vi "GetPirticleResultNames.vi"(7 "ProjectName":string="Prj", 9 "Selected Particle Report":T1(array[cluster])=[{"Area"=25.0, "Number of Holes"=0.0, "Bounding Rect"={"Left"=86.0, "Top"=0.0, "Right"=95.0, "Bottom"=7.0}, "Center of Mass"={"X"=89.88, "Y"=2.56}, "Orientation"=35.64802944169076, "Dimensions"={"Width"=9.0, "Height"=7.0}}, {"Area"=86262.0, "Number of Holes"=23.0, "Bounding Rect"={"Left"=0.0, "Top"=0.0, "Right"=463.0, "Bottom"=400.0}, "Center of Mass"={"X"=231.6348565996615, "Y"=215.4975423709165}, "Orientation"=163.33264135410136, "Dimensions"={"Width"=463.0, "Height"=400.0}}, {"Area"=1.0, "Number of Holes"=0.0, "Bounding Rect"={"Left"=412.0, "Top"=1.0, "Right"=413.0, "Bottom"=2.0}, "Center of Mass"={"X"=412.0, "Y"=1.0}, "Orientation"=-0.0, "Dimensions"={"Width"=1.0, "Height"=1.0}}, {"Area"=764.0, "Number of Holes"=1.0, "Bounding Rect"={"Left"=400.0, "Top"=1.0, "Right"=429.0, "Bottom"=38.0}, "Center of Mass"={"X"=414.1609947643979, "Y"=19.994764397905758}, "Orientation"=91.15464026101695, "Dimensions"={"Width"=29.0, "Height"=37.0}}, {"Area"=59.0, "Number of Holes"=0.0, "Bounding Rect"={"Left"=310.0, "Top"=6.0, "Right"=340.0, "Bottom"=29.0}, "Center of Mass"={"X"=326.50847457627117, "Y"=15.610169491525424}, "Orientation"=141.9692279302436, "Dimensions"={"Width"=30.0, "Height"=23.0}}, {"Area"=11.0, "Number of Holes"=0.0, "Bounding Rect"={"Left"=0.0, "Top"=7.0, "Right"=8.0, "Bottom"=12.0}, "Center of Mass"={"X"=3.090909090909091, "Y"=9.0}, "Orientation"=154.0962999034186, "Dimensions"={"Width"=8.0, "Height"=5.0}}, {"Area"=8.0, "Number of Holes"=0.0, "Bounding Rect"={"Left"=10.0, "Top"=12.0, "Right"=18.0, "Bottom"=15.0}, "Center of Mass"={"X"=13.5, "Y"=13.125}, "Orientation"=161.9863133074482, "Dimensions"={"Width"=8.0, "Height"=3.0}}, {"Area"=2191.0, "Number of Holes"=0.0, "Bounding Rect"={"Left"=108.0, "Top"=12.0, "Right"=160.0, "Bottom"=73.0}, "Center of Mass"={"X"=132.4596074851666, "Y"=44.30716567777271}, "Orientation"=94.97370367521454, "Dimensions"={"Width"=52.0, "Height"=61.0}}, {"Area"=18.0, "Number of Holes"=0.0, "Bounding Rect"={"Left"=136.0, "Top"=12.0, "Right"=150.0, "Bottom"=18.0}, "Center of Mass"={"X"=142.94444444444446, "Y"=13.833333333333334}, "Orientation"=159.1562056734768, "Dimensions"={"Width"=14.0, "Height"=6.0}}, {"Area"=4659.0, "Number of Holes"=2.0, "Bounding Rect"={"Left"=266.0, "Top"=12.0, "Right"=345.0, "Bottom"=101.0}, "Center of Mass"={"X"=303.5157759175789, "Y"=58.89869070616012}, "Orientation"=93.68626534635163, "Dimensions"={"Width"=79.0, "Height"=89.0}}, {"Area"=12.0, "Number of Holes"=0.0, "Bounding Rect"={"Left"=19.0, "Top"=14.0, "Right"=29.0, "Bottom"=17.0}, "Center of Mass"={"X"=23.083333333333332, "Y"=15.416666666666666}, "Orientation"=169.41797481154816, "Dimensions"={"Width"=10.0, "Height"=3.0}}, {"Area"=6.0, "Number of Holes"=0.0, "Bounding Rect"={"Left"=32.0, "Top"=17.0, "Right"=38.0, "Bottom"=18.0}, "Center of Mass"={"X"=34.5, "Y"=17.0}, "Orientation"=-0.0, "Dimensions"={"Width"=6.0, "Height"=1.0}}, {"Area"=1.0, "Number of Holes"=0.0, "Bounding Rect"={"Left"=40.0, "Top"=17.0, "Right"=41.0, "Bottom"=18.0}, "Center of Mass"={"X"=40.0, "Y"=17.0}, "Orientation"=-0.0, "Dimensions"={"Width"=1.0, "Height"=1.0}}, {"Area"=1.0, "Number of Holes"=0.0, "Bounding Rect"={"Left"=326.0, "Top"=23.0, "Right"=327.0, "Bottom"=24.0}, "Center of Mass"={"X"=326.0, "Y"=23.0}, "Orientation"=-0.0, "Dimensions"={"Width"=1.0, "Height"=1.0}}, {"Area"=72.0, "Number of Holes"=2.0, "Bounding Rect"={"Left"=388.0, "Top"=35.0, "Right"=410.0, "Bottom"=55.0}, "Center of Mass"={"X"=397.8888888888889, "Y"=46.52777777777778}, "Orientation"=136.8853757704328, "Dimensions"={"Width"=22.0, "Height"=20.0}}, {"Area"=2.0, "Number of Holes"=0.0, "Bounding Rect"={"Left"=342.0, "Top"=36.0, "Right"=343.0, "Bottom"=38.0}, "Center of Mass"={"X"=342.0, "Y"=36.5}, "Orientation"=90.0, "Dimensions"={"Width"=1.0, "Height"=2.0}}, {"Area"=1.0, "Number of Holes"=0.0, "Bounding Rect"={"Left"=396.0, "Top"=49.0, "Right"=397.0, "Bottom"=50.0}, "Center of Mass"={"X"=396.0, "Y"=49.0}, "Orientation"=-0.0, "Dimensions"={"Width"=1.0, "Height"=1.0}}, {"Area"=2.0, "Number of Holes"=0.0, "Bounding Rect"={"Left"=411.0, "Top"=54.0, "Right"=413.0, "Bottom"=55.0}, "Center of Mass"={"X"=411.5, "Y"=54.0}, "Orientation"=-0.0, "Dimensions"={"Width"=2.0, "Height"=1.0}}, {"Area"=86.0, "Number of Holes"=0.0, "Bounding Rect"={"Left"=457.0, "Top"=74.0, "Right"=463.0, "Bottom"=96.0}, "Center of Mass"={"X"=460.2674418604651, "Y"=84.55813953488372}, "Orientation"=89.65892383367937, "Dimensions"={"Width"=6.0, "Height"=22.0}}, {"Area"=1300.0, "Number of Holes"=0.0, "Bounding Rect"={"Left"=30.0, "Top"=82.0, "Right"=67.0, "Bottom"=127.0}, "Center of Mass"={"X"=48.050769230769234, "Y"=104.12153846153846}, "Orientation"=84.17144755534598, "Dimensions"={"Width"=37.0, "Height"=45.0}}, {"Area"=1.0, "Number of Holes"=0.0, "Bounding Rect"={"Left"=450.0, "Top"=105.0, "Right"=451.0, "Bottom"=106.0}, "Center of Mass"={"X"=450.0, "Y"=105.0}, "Orientation"=-0.0, "Dimensions"={"Width"=1.0, "Height"=1.0}}, {"Area"=3.0, "Number of Holes"=0.0, "Bounding Rect"={"Left"=243.0, "Top"=124.0, "Right"=245.0, "Bottom"=126.0}, "Center of Mass"={"X"=243.66666666666666, "Y"=124.33333333333333}, "Orientation"=135.00000000000014, "Dimensions"={"Width"=2.0, "Height"=2.0}}, {"Area"=28.0, "Number of Holes"=0.0, "Bounding Rect"={"Left"=271.0, "Top"=127.0, "Right"=293.0, "Bottom"=136.0}, "Center of Mass"={"X"=281.39285714285717, "Y"=131.39285714285714}, "Orientation"=158.88118737593115, "Dimensions"={"Width"=22.0, "Height"=9.0}}, {"Area"=4.0, "Number of Holes"=0.0, "Bounding Rect"={"Left"=250.0, "Top"=128.0, "Right"=253.0, "Bottom"=130.0}, "Center of Mass"={"X"=251.0, "Y"=128.5}, "Orientation"=148.282525588539, "Dimensions"={"Width"=3.0, "Height"=2.0}}, {"Area"=4.0, "Number of Holes"=0.0, "Bounding Rect"={"Left"=255.0, "Top"=132.0, "Right"=258.0, "Bottom"=134.0}, "Center of Mass"={"X"=256.0, "Y"=132.5}, "Orientation"=148.282525588539, "Dimensions"={"Width"=3.0, "Height"=2.0}}, {"Area"=2.0, "Number of Holes"=0.0, "Bounding Rect"={"Left"=260.0, "Top"=136.0, "Right"=262.0, "Bottom"=138.0}, "Center of Mass"={"X"=260.5, "Y"=136.5}, "Orientation"=135.0, "Dimensions"={"Width"=2.0, "Height"=2.0}}, {"Area"=1.0, "Number of Holes"=0.0, "Bounding Rect"={"Left"=300.0, "Top"=136.0, "Right"=301.0, "Bottom"=137.0}, "Center of Mass"={"X"=300.0, "Y"=136.0}, "Orientation"=-0.0, "Dimensions"={"Width"=1.0, "Height"=1.0}}, {"Area"=6.0, "Number of Holes"=0.0, "Bounding Rect"={"Left"=263.0, "Top"=139.0, "Right"=269.0, "Bottom"=145.0}, "Center of Mass"={"X"=265.5, "Y"=141.5}, "Orientation"=135.0, "Dimensions"={"Width"=6.0, "Height"=6.0}}, {"Area"=4.0, "Number of Holes"=0.0, "Bounding Rect"={"Left"=296.0, "Top"=139.0, "Right"=299.0, "Bottom"=141.0}, "Center of Mass"={"X"=297.25, "Y"=139.25}, "Orientation"=161.56505117707798, "Dimensions"={"Width"=3.0, "Height"=2.0}}, {"Area"=1.0, "Number of Holes"=0.0, "Bounding Rect"={"Left"=269.0, "Top"=146.0, "Right"=270.0, "Bottom"=147.0}, "Center of Mass"={"X"=269.0, "Y"=146.0}, "Orientation"=-0.0, "Dimensions"={"Width"=1.0, "Height"=1.0}}, {"Area"=3.0, "Number of Holes"=0.0, "Bounding Rect"={"Left"=271.0, "Top"=148.0, "Right"=273.0, "Bottom"=151.0}, "Center of Mass"={"X"=271.3333333333333, "Y"=149.0}, "Orientation"=118.15496623701016, "Dimensions"={"Width"=2.0, "Height"=3.0}}, {"Area"=2795.0, "Number of Holes"=2.0, "Bounding Rect"={"Left"=375.0, "Top"=149.0, "Right"=427.0, "Bottom"=220.0}, "Center of Mass"={"X"=400.8608228980322, "Y"=184.37352415026834}, "Orientation"=84.46336335814708, "Dimensions"={"Width"=52.0, "Height"=71.0}}, {"Area"=6024.0, "Number of Holes"=9.0, "Bounding Rect"={"Left"=176.0, "Top"=152.0, "Right"=254.0, "Bottom"=252.0}, "Center of Mass"={"X"=211.63097609561754, "Y"=201.42861885790174}, "Orientation"=84.84991716022375, "Dimensions"={"Width"=78.0, "Height"=100.0}}, {"Area"=1.0, "Number of Holes"=0.0, "Bounding Rect"={"Left"=275.0, "Top"=154.0, "Right"=276.0, "Bottom"=155.0}, "Center of Mass"={"X"=275.0, "Y"=154.0}, "Orientation"=-0.0, "Dimensions"={"Width"=1.0, "Height"=1.0}}, {"Area"=2.0, "Number of Holes"=0.0, "Bounding Rect"={"Left"=462.0, "Top"=209.0, "Right"=463.0, "Bottom"=211.0}, "Center of Mass"={"X"=462.0, "Y"=209.5}, "Orientation"=90.0, "Dimensions"={"Width"=1.0, "Height"=2.0}}, {"Area"=1.0, "Number of Holes"=0.0, "Bounding Rect"={"Left"=460.0, "Top"=214.0, "Right"=461.0, "Bottom"=215.0}, "Center of Mass"={"X"=460.0, "Y"=214.0}, "Orientation"=-0.0, "Dimensions"={"Width"=1.0, "Height"=1.0}}, {"Area"=2.0, "Number of Holes"=0.0, "Bounding Rect"={"Left"=459.0, "Top"=216.0, "Right"=460.0, "Bottom"=218.0}, "Center of Mass"={"X"=459.0, "Y"=216.5}, "Orientation"=90.0, "Dimensions"={"Width"=1.0, "Height"=2.0}}, {"Area"=3.0, "Number of Holes"=0.0, "Bounding Rect"={"Left"=249.0, "Top"=220.0, "Right"=251.0, "Bottom"=223.0}, "Center of Mass"={"X"=249.66666666666666, "Y"=221.0}, "Orientation"=61.84503376298985, "Dimensions"={"Width"=2.0, "Height"=3.0}}, {"Area"=1243.0, "Number of Holes"=2.0, "Bounding Rect"={"Left"=26.0, "Top"=222.0, "Right"=62.0, "Bottom"=266.0}, "Center of Mass"={"X"=43.17940466613033, "Y"=243.51729686242962}, "Orientation"=85.94368880614128, "Dimensions"={"Width"=36.0, "Height"=44.0}}, {"Area"=3.0, "Number of Holes"=0.0, "Bounding Rect"={"Left"=248.0, "Top"=224.0, "Right"=250.0, "Bottom"=227.0}, "Center of Mass"={"X"=248.33333333333334, "Y"=225.0}, "Orientation"=61.84503376298985, "Dimensions"={"Width"=2.0, "Height"=3.0}}, {"Area"=1.0, "Number of Holes"=0.0, "Bounding Rect"={"Left"=62.0, "Top"=237.0, "Right"=63.0, "Bottom"=238.0}, "Center of Mass"={"X"=62.0, "Y"=237.0}, "Orientation"=-0.0, "Dimensions"={"Width"=1.0, "Height"=1.0}}, {"Area"=1.0, "Number of Holes"=0.0, "Bounding Rect"={"Left"=63.0, "Top"=241.0, "Right"=64.0, "Bottom"=242.0}, "Center of Mass"={"X"=63.0, "Y"=241.0}, "Orientation"=-0.0, "Dimensions"={"Width"=1.0, "Height"=1.0}}, {"Area"=25.0, "Number of Holes"=0.0, "Bounding Rect"={"Left"=60.0, "Top"=277.0, "Right"=78.0, "Bottom"=285.0}, "Center of Mass"={"X"=68.52, "Y"=279.96}, "Orientation"=21.66201240397291, "Dimensions"={"Width"=18.0, "Height"=8.0}}, {"Area"=2.0, "Number of Holes"=0.0, "Bounding Rect"={"Left"=57.0, "Top"=285.0, "Right"=59.0, "Bottom"=287.0}, "Center of Mass"={"X"=57.5, "Y"=285.5}, "Orientation"=45.0, "Dimensions"={"Width"=2.0, "Height"=2.0}}, {"Area"=1575.0, "Number of Holes"=0.0, "Bounding Rect"={"Left"=302.0, "Top"=285.0, "Right"=345.0, "Bottom"=337.0}, "Center of Mass"={"X"=321.4095238095238, "Y"=308.74603174603175}, "Orientation"=73.7943685874199, "Dimensions"={"Width"=43.0, "Height"=52.0}}, {"Area"=4853.0, "Number of Holes"=6.0, "Bounding Rect"={"Left"=54.0, "Top"=304.0, "Right"=130.0, "Bottom"=388.0}, "Center of Mass"={"X"=91.93962497424273, "Y"=344.35854110859265}, "Orientation"=86.14198788768665, "Dimensions"={"Width"=76.0, "Height"=84.0}}, {"Area"=28.0, "Number of Holes"=0.0, "Bounding Rect"={"Left"=323.0, "Top"=332.0, "Right"=338.0, "Bottom"=341.0}, "Center of Mass"={"X"=330.57142857142856, "Y"=336.64285714285717}, "Orientation"=29.47782205630064, "Dimensions"={"Width"=15.0, "Height"=9.0}}, {"Area"=3.0, "Number of Holes"=0.0, "Bounding Rect"={"Left"=312.0, "Top"=366.0, "Right"=315.0, "Bottom"=367.0}, "Center of Mass"={"X"=313.0, "Y"=366.0}, "Orientation"=-0.0, "Dimensions"={"Width"=3.0, "Height"=1.0}}, {"Area"=1.0, "Number of Holes"=0.0, "Bounding Rect"={"Left"=436.0, "Top"=396.0, "Right"=437.0, "Bottom"=397.0}, "Center of Mass"={"X"=436.0, "Y"=396.0}, "Orientation"=-0.0, "Dimensions"={"Width"=1.0, "Height"=1.0}}, {"Area"=1.0, "Number of Holes"=0.0, "Bounding Rect"={"Left"=434.0, "Top"=397.0, "Right"=435.0, "Bottom"=398.0}, "Center of Mass"={"X"=434.0, "Y"=397.0}, "Orientation"=-0.0, "Dimensions"={"Width"=1.0, "Height"=1.0}}, {"Area"=36.0, "Number of Holes"=0.0, "Bounding Rect"={"Left"=318.0, "Top"=398.0, "Right"=340.0, "Bottom"=400.0}, "Center of Mass"={"X"=328.5, "Y"=398.6111111111111}, "Orientation"=-0.0, "Dimensions"={"Width"=22.0, "Height"=2.0}}, {"Area"=8.0, "Number of Holes"=0.0, "Bounding Rect"={"Left"=427.0, "Top"=398.0, "Right"=433.0, "Bottom"=400.0}, "Center of Mass"={"X"=429.75, "Y"=398.625}, "Orientation"=11.525650458236512, "Dimensions"={"Width"=6.0, "Height"=2.0}}], 10 "Analysis_Particle_Parameter":T2={"Selected Particle"=0, "Connectivity 4/8 (8)"=TRUE, "MaxParticle"=0}, 11 "ROI_Name":string="ROI1") -> (3 "ResultNames":string[](array[string]))   [LabVIEW 2019]
uses:
  Controls/Particle/Analysis_Particle_Result.ctl
  Controls/Particle/Analysis_Particle_Parameter.ctl
panel:
  in  "Analysis_Particle_Result":T3 {"Selected Particle Report"."Orientation" format="%.2f"; "Selected Particle Report"."Center of Mass"."Y" format="%.2f"; "Selected Particle Report"."Center of Mass"."X" format="%.2f"}
  out "error out":errorcluster
  in  "error in (no error)":errorcluster
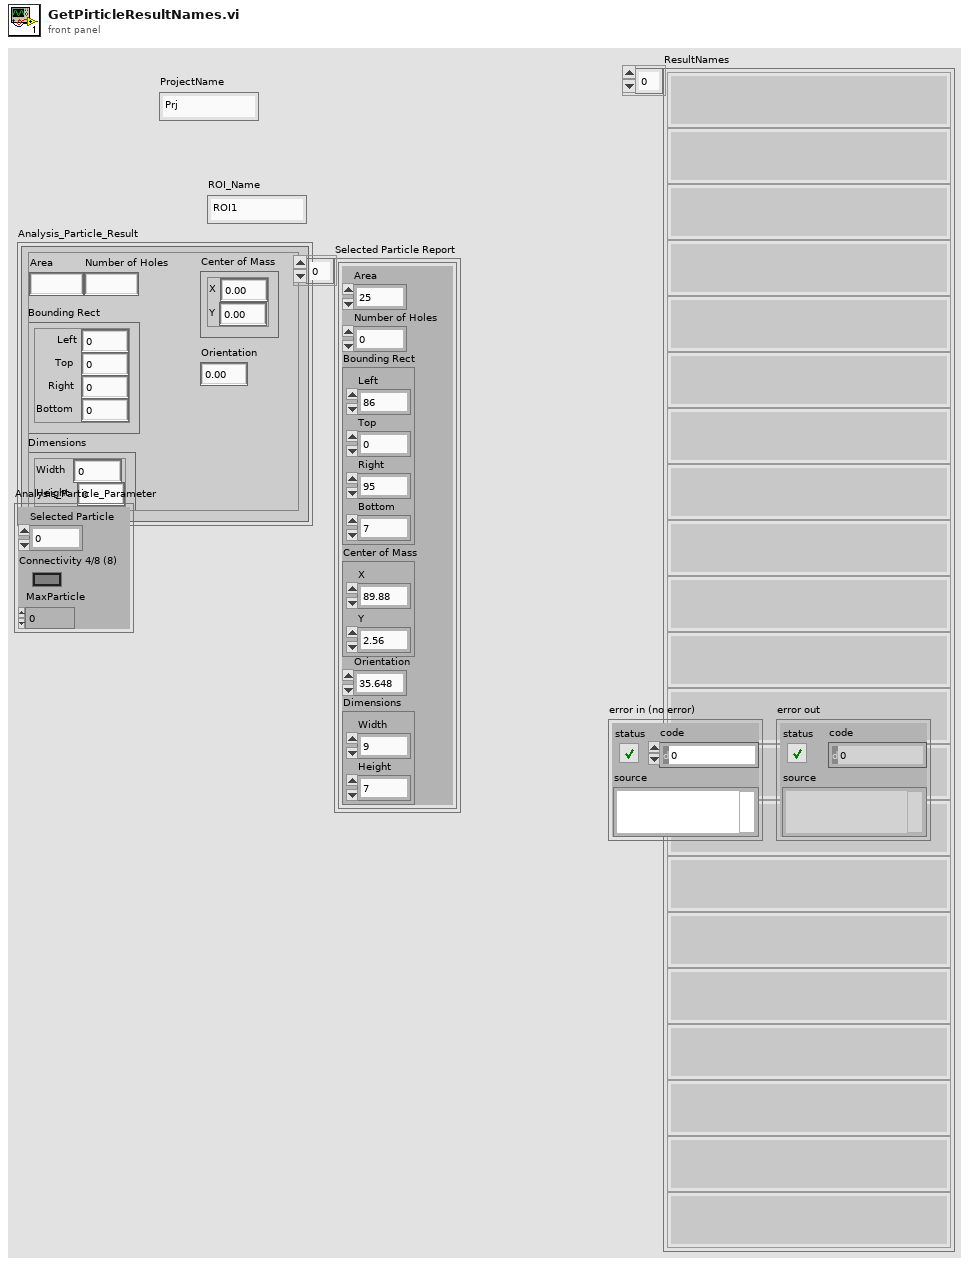
[diagram p1: front panel]
types:
  T1 = cluster{"Area":dbl, "Number of Holes":dbl, "Bounding Rect":cluster{"Left":dbl, "Top":dbl, "Right":dbl, "Bottom":dbl}, "Center of Mass":cluster{"X":dbl, "Y":dbl}, "Orientation":dbl, "Dimensions":cluster{"Width":dbl, "Height":dbl}}[]
  T2 = typedef "Analysis_Particle_Parameter.ctl" = cluster{"Selected Particle":i32, "Connectivity 4/8 (8)":bool, "MaxParticle":i32}
  T3 = typedef "Analysis_Particle_Result.ctl" = cluster{"Selected Particle Report":cluster{"Area":dbl, "Number of Holes":dbl, "Bounding Rect":cluster{"Left":dbl, "Top":dbl, "Right":dbl, "Bottom":dbl}, "Center of Mass":cluster{"X":dbl, "Y":dbl}, "Orientation":dbl, "Dimensions":cluster{"Width":dbl, "Height":dbl}}}
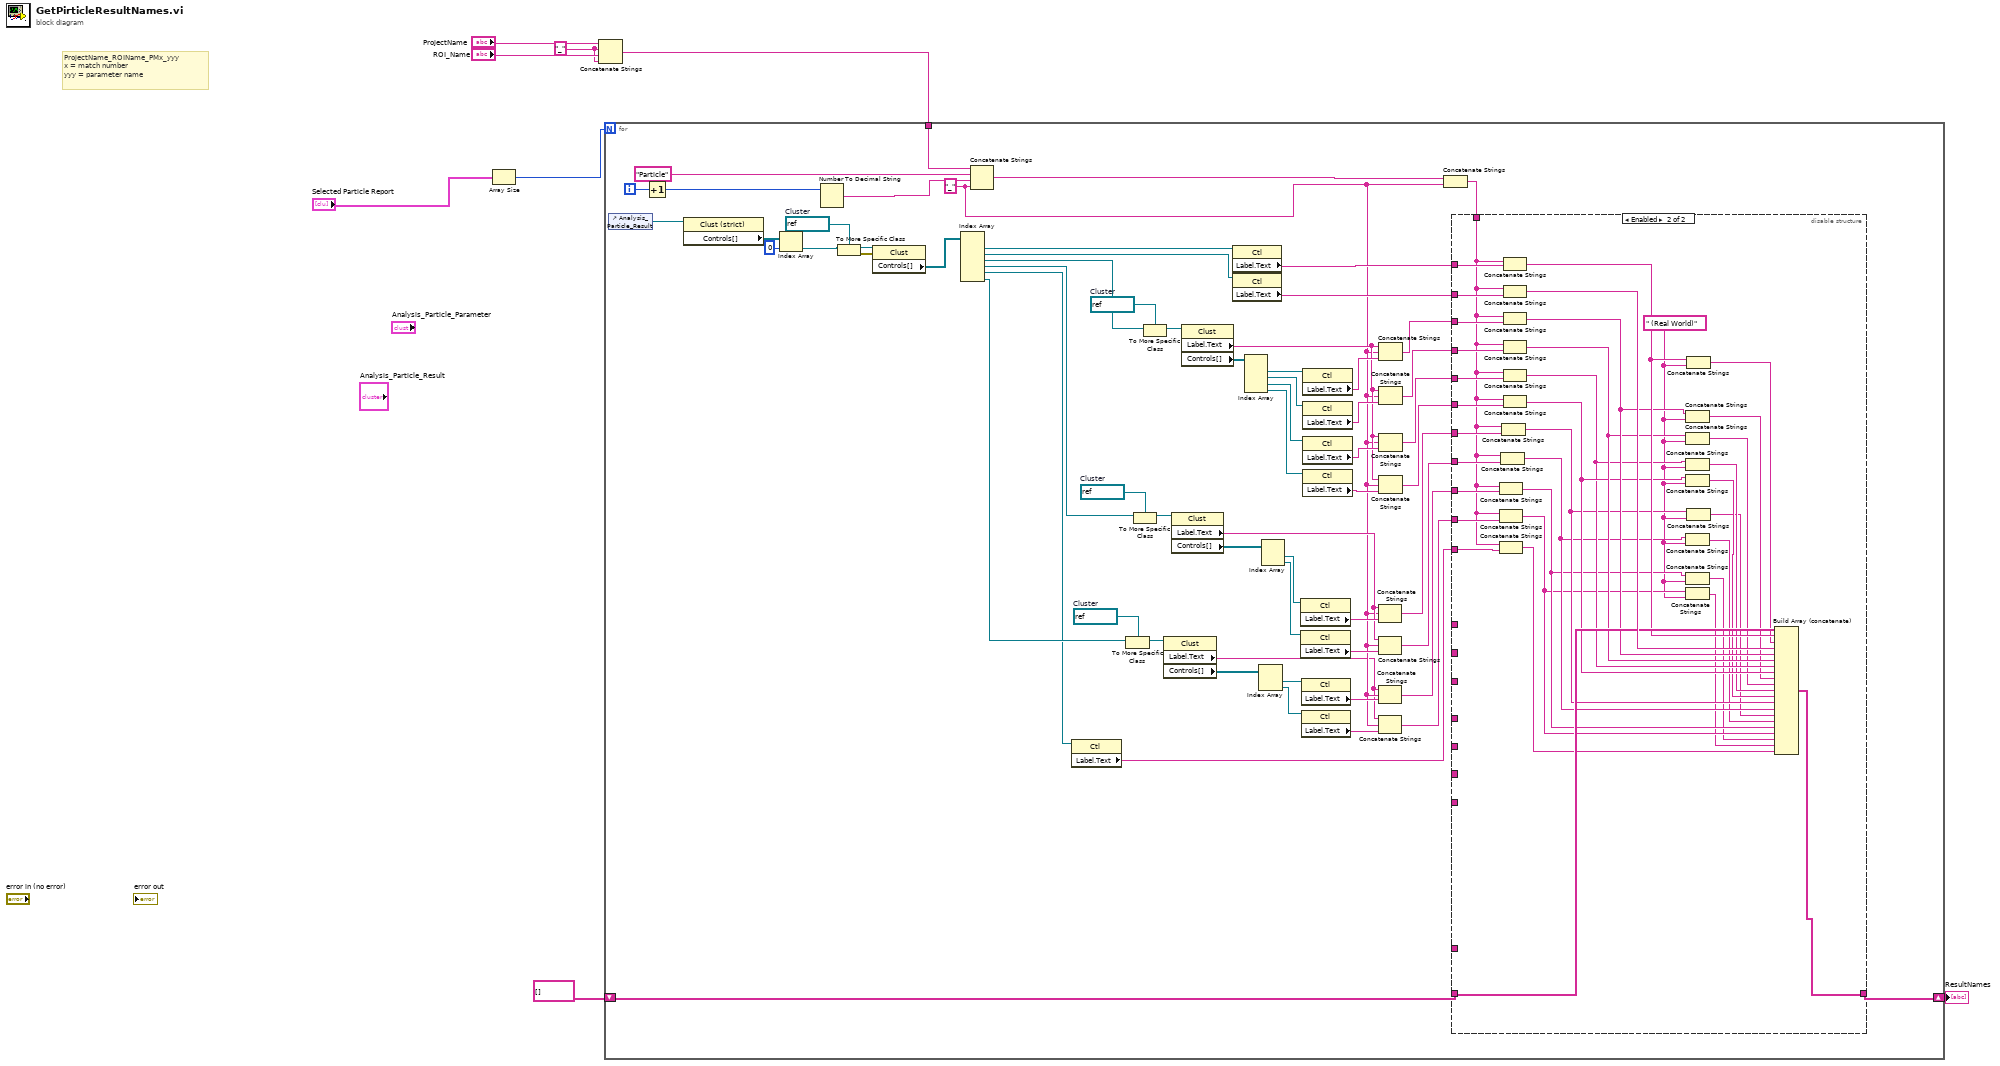
[diagram p0: block diagram]
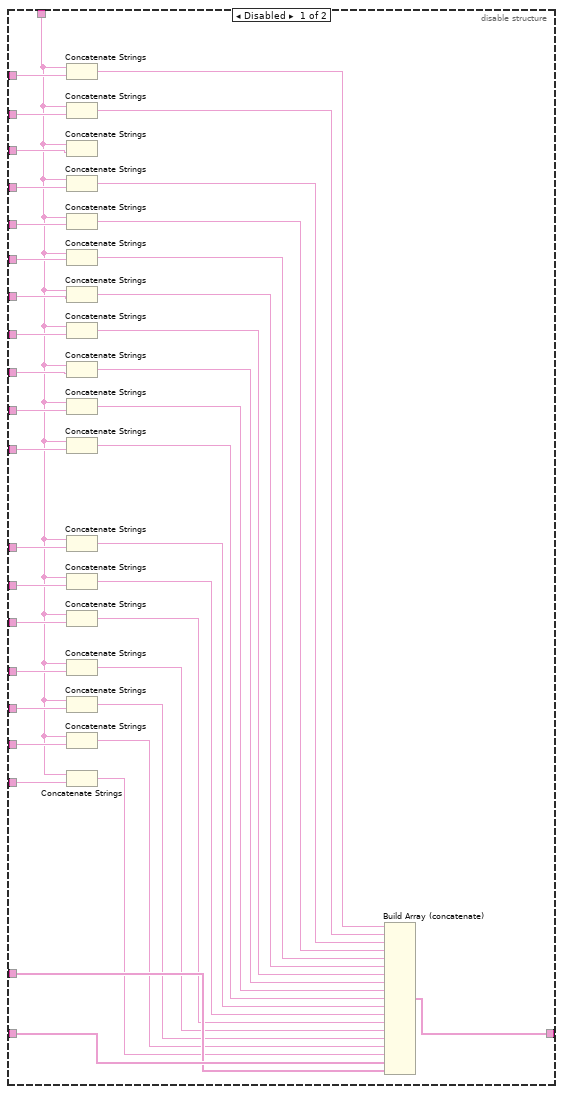
[diagram p2: hidden frame]
diagram:
  w6 = "_" ("string")
  # "ProjectName_ROIName_PMx_yyy\nx = match number\nyyy = parameter name"
  n1 = Array Size(array="Selected Particle Report") -> (size(s)=w2:i32)
  n2 = Concatenate Strings("ProjectName", w6, "ROI_Name", w6) -> (w5:string)
  n3 = for {
    N: w2 -> [_]
    tunnel: w5 -> [w70]
    shift-right: [w59] -> w3
    shift-left: string[] [] -> [w66]
    i -> [w67]
    w16 = "_" ("string")
    w14 = refnum<vi> refnum  # Cluster
    w22 = refnum<vi> refnum  # Cluster
    w49 = refnum<vi> refnum  # Cluster
    w55 = refnum<vi> refnum  # Cluster
    n4 = control-ref of="Analysis_Particle_Result"() -> (w51:refnum<vi>)
    n5 = Increment(x=w67) -> (x+1=w71:i32)
    n6 = property class="Clust (strict)"(reference=w51) -> ("Controls[]"=w58:refnum<vi>[])  [unwired: 1 in, 2 out]
    n7 = Index Array(array=w58, index=0) -> (element=w56:refnum<vi>)
    n8 = Number To Decimal String(number=w71) -> (decimal integer string=w69:string)  [unwired: 1 in]
    n9 = To More Specific Class(target class=w55, reference=w56) -> (specific class reference=w54:refnum<vi>, error out=w53:errorcluster)  [unwired: 1 in]
    n10 = property class="Clust"(reference=w54, error in=w53) -> ("Controls[]"=w52:refnum<vi>[])  [unwired: 2 out]
    n11 = Index Array(array=w52) -> (element #1=w65:refnum<vi>, element #2=w64:refnum<vi>, element #3=w50:refnum<vi>, element #4=w34:refnum<vi>, element #5=w11:refnum<vi>, element #6=w12:refnum<vi>)  [unwired: 6 in]
    n12 = Concatenate Strings(w70, "Particle" ("string"), w69, w16) -> (w63:string)
    n13 = property class="Ctl"(reference=w11) -> ("Label.Text"=w24:string)  [unwired: 1 in, 2 out]
    n14 = To More Specific Class(target class=w14, reference=w12) -> (specific class reference=w13:refnum<vi>)  [unwired: 1 in, 1 out]
    n15 = To More Specific Class(target class=w22, reference=w34) -> (specific class reference=w23:refnum<vi>)  [unwired: 1 in, 1 out]
    n16 = To More Specific Class(target class=w49, reference=w50) -> (specific class reference=w48:refnum<vi>)  [unwired: 1 in, 1 out]
    n17 = property class="Clust"(reference=w13) -> ("Label.Text"=w15:string, "Controls[]"=w20:refnum<vi>[])  [unwired: 1 in, 2 out]
    n18 = property class="Clust"(reference=w23) -> ("Label.Text"=w17:string, "Controls[]"=w21:refnum<vi>[])  [unwired: 1 in, 2 out]
    n19 = property class="Clust"(reference=w48) -> ("Label.Text"=w29:string, "Controls[]"=w43:refnum<vi>[])  [unwired: 1 in, 2 out]
    n20 = property class="Ctl"(reference=w65) -> ("Label.Text"=w62:string)  [unwired: 1 in, 2 out]
    n21 = property class="Ctl"(reference=w64) -> ("Label.Text"=w61:string)  [unwired: 1 in, 2 out]
    n22 = Index Array(array=w43) -> (element #1=w47:refnum<vi>, element #2=w46:refnum<vi>, element #3=w45:refnum<vi>, element #4=w44:refnum<vi>)  [unwired: 4 in]
    n23 = Index Array(array=w20) -> (element #1=w10:refnum<vi>, element #2=w9:refnum<vi>)  [unwired: 2 in]
    n24 = Index Array(array=w21) -> (element #1=w19:refnum<vi>, element #2=w18:refnum<vi>)  [unwired: 2 in]
    n25 = property class="Ctl"(reference=w19) -> ("Label.Text"=w33:string)  [unwired: 1 in, 2 out]
    n26 = property class="Ctl"(reference=w18) -> ("Label.Text"=w31:string)  [unwired: 1 in, 2 out]
    n27 = property class="Ctl"(reference=w10) -> ("Label.Text"=w32:string)  [unwired: 1 in, 2 out]
    n28 = property class="Ctl"(reference=w9) -> ("Label.Text"=w30:string)  [unwired: 1 in, 2 out]
    n29 = property class="Ctl"(reference=w47) -> ("Label.Text"=w42:string)  [unwired: 1 in, 2 out]
    n30 = property class="Ctl"(reference=w46) -> ("Label.Text"=w40:string)  [unwired: 1 in, 2 out]
    n31 = property class="Ctl"(reference=w45) -> ("Label.Text"=w39:string)  [unwired: 1 in, 2 out]
    n32 = property class="Ctl"(reference=w44) -> ("Label.Text"=w38:string)  [unwired: 1 in, 2 out]
    n33 = Concatenate Strings(w17, w16, w33) -> (w28:string)
    n34 = Concatenate Strings(w17, w16, w31) -> (w27:string)
    n35 = Concatenate Strings(w15, w16, w32) -> (w26:string)
    n36 = Concatenate Strings(w15, w16, w30) -> (w25:string)
    n37 = Concatenate Strings(w29, w16, w42) -> (w41:string)
    n38 = Concatenate Strings(w29, w16, w40) -> (w37:string)
    n39 = Concatenate Strings(w29, w16, w39) -> (w36:string)
    n40 = Concatenate Strings(w29, w16, w38) -> (w35:string)
    n41 = Concatenate Strings(w63, w16) -> (w60:string)
    n42 = disable-structure shown="Enabled" {
      disable-tunnel: w66 -> [w110 w142]
      disable-tunnel: _ -> [w109 _]
      disable-tunnel: w62 -> [w108 w144]
      disable-tunnel: w61 -> [w107 w145]
      disable-tunnel: w37 -> [w106 w140]
      disable-tunnel: w36 -> [w105 w139]
      disable-tunnel: w60 -> [w84 w132]
      disable-tunnel: [w101 w129] -> w59
      disable-tunnel: w35 -> [w99 w138]
      disable-tunnel: w41 -> [w97 w141]
      disable-tunnel: w28 -> [w96 w137]
      disable-tunnel: w27 -> [w95 w136]
      disable-tunnel: w26 -> [w94 w135]
      disable-tunnel: w25 -> [w93 w134]
      disable-tunnel: w24 -> [w92 w133]
      disable-tunnel: _ -> [w91 _]
      disable-tunnel: _ -> [w90 _]
      disable-tunnel: _ -> [w89 _]
      disable-tunnel: _ -> [w88 _]
      disable-tunnel: _ -> [w87 _]
      disable-tunnel: _ -> [w86 _]
      disable-tunnel: _ -> [w85 _]
      frame Disabled {
        n43 = Concatenate Strings(w84, w108) -> (w104:string)
        n44 = Concatenate Strings(w84, w107) -> (w103:string)
        n45 = Concatenate Strings(w84, w97) -> ()  [unwired: 1 out]
        n46 = Concatenate Strings(w84, w106) -> (w102:string)
        n47 = Concatenate Strings(w84, w105) -> (w100:string)
        n48 = Concatenate Strings(w84, w99) -> (w98:string)
        n49 = Concatenate Strings(w84, w96) -> (w83:string)
        n50 = Concatenate Strings(w84, w95) -> (w82:string)
        n51 = Concatenate Strings(w84, w94) -> (w81:string)
        n52 = Concatenate Strings(w84, w93) -> (w80:string)
        n53 = Concatenate Strings(w84, w92) -> (w79:string)
        n54 = Concatenate Strings(w84, w91) -> (w78:string)
        n55 = Concatenate Strings(w84, w90) -> (w77:string)
        n56 = Concatenate Strings(w84, w89) -> (w76:string)
        n57 = Concatenate Strings(w84, w88) -> (w75:string)
        n58 = Concatenate Strings(w84, w87) -> (w74:string)
        n59 = Concatenate Strings(w84, w86) -> (w73:string)
        n60 = Concatenate Strings(w84, w85) -> (w72:string)
        n61 = Build Array (concatenate)(w104, w103, w102, w100, w98, w83, w82, w81, w80, w79, w78, w77, w76, w75, w74, w73, w72, w110, w109) -> (w101:string[])
      }
      frame Enabled {
        w115 = " (Real World)" ("string")
        n62 = Concatenate Strings(w132, w135) -> (w117:string)
        n63 = Concatenate Strings(w132, w134) -> (w116:string)
        n64 = Concatenate Strings(w132, w133) -> (w131:string)
        n65 = Concatenate Strings(w132, w136) -> (w118:string)
        n66 = Concatenate Strings(w132, w137) -> (w119:string)
        n67 = Concatenate Strings(w132, w144) -> (w130:string)
        n68 = Concatenate Strings(w132, w145) -> (w143:string)
        n69 = Concatenate Strings(w132, w141) -> (w127:string)
        n70 = Concatenate Strings(w132, w140) -> (w126:string)
        n71 = Concatenate Strings(w132, w139) -> (w124:string)
        n72 = Concatenate Strings(w132, w138) -> (w125:string)
        n73 = Concatenate Strings(w127, w115) -> (w123:string)
        n74 = Concatenate Strings(w126, w115) -> (w122:string)
        n75 = Concatenate Strings(w124, w115) -> (w121:string)
        n76 = Concatenate Strings(w125, w115) -> (w120:string)
        n77 = Concatenate Strings(w118, w115) -> (w113:string)
        n78 = Concatenate Strings(w117, w115) -> (w112:string)
        n79 = Concatenate Strings(w116, w115) -> (w111:string)
        n80 = Concatenate Strings(w130, w115) -> (w128:string)
        n81 = Concatenate Strings(w119, w115) -> (w114:string)
        n82 = Build Array (concatenate)(w142, w130, w128, w143, w127, w126, w124, w125, w123, w122, w121, w120, w119, w118, w114, w113, w117, w116, w112, w111, w131) -> (w129:string[])
      }
    }
  }
  "ResultNames" <- w3
